vi "Initialize.vi"(8 "error in (no error)":errorcluster, 9 "VISA Com Port":refnum<visa-resource-name>, 10 "Serial Device Brand":T1, 11 "NXP in":refnum<class "NXP.lvclass">) -> (0 "error out":errorcluster, 3 "NXP out":refnum<class "NXP.lvclass">)   [LabVIEW 2020, in "NXP.lvclass"]
uses:
  NXP.lvclass
  Controles/Brand combobox.ctl
  <vilib>/Instr/_visa.llb/VISA Configure Serial Port (Instr).vi
  Abstract/Serial device/Serial device.lvclass
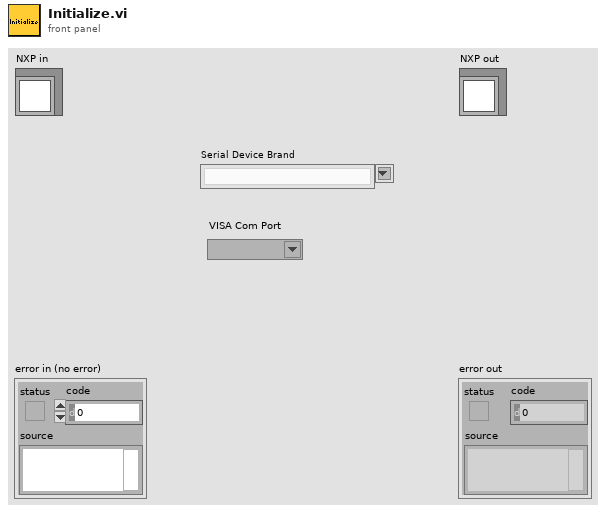
[diagram p1: front panel]
types:
  T1 = typedef "Serial device.lvclass/Brand combobox.ctl" = string
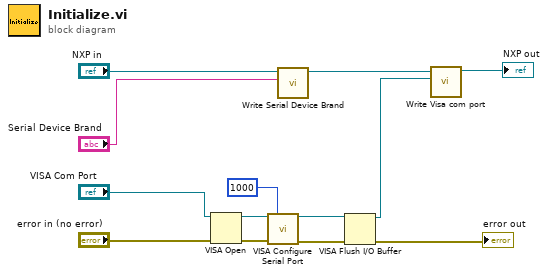
[diagram p0: block diagram]
diagram:
  n1 = VISA Open(error in (no error)="error in (no error)", VISA resource name="VISA Com Port") -> (VISA resource name=w9:refnum<visa-resource-name>, error out=w8:errorcluster)  [unwired: 3 in]
  n2 = call-poly "VISA Configure Serial Port"("VISA resource name"=w9, "timeout (10sec)"=u32 1000, "error in (no error)"=w8) -> ("VISA resource name out"=w7:refnum<visa-resource-name>, "error out"=w6:errorcluster)  [unwired: 11 in]
  n3 = call-dynamic "Write Serial Device Brand.vi"("Serial Device Brand"="Serial Device Brand", "Serial device in"="NXP in") -> ("Serial device out"=w12:refnum<class "NXP.lvclass">)  [unwired: 8 in, 1 out]
  n4 = VISA Flush I/O Buffer(VISA resource name=w7, error in (no error)=w6) -> (VISA resource name out=w2:refnum<visa-resource-name>, error out=→"error out":errorcluster)  [unwired: 1 in]
  n5 = call-dynamic "Write Visa com port.vi"("Visa com port"=w2, "Serial device in"=w12) -> ("Serial device out"=→"NXP out":refnum<class "NXP.lvclass">)  [unwired: 8 in, 1 out]
